vi "Find MBR of Polygon.vi"(0 "Overlay Ref":refnum<k24>, 11 "error in (no error)":errorcluster) -> (3 "Points of Polygon":T1[](array[typedef]) {"Latitude" format="%#_10g"; "Longitude" format="%#_10g"}, 4 "Min Lat":dbl format="%#.6g", 6 "Min Lon":dbl format="%#.6g", 8 "Max Lat":dbl format="%#.6g", 10 "Max Lon":dbl format="%#.6g", 14 "Bearing Between First two Points":dbl, 15 "error out":errorcluster)   [LabVIEW 2014]
uses:
  C:/Robotic Systems/Products/AgFalcon/Software/Ground Station/Data/Mapping DLL/GMap.NET.WindowsForms.dll
  Data/Mapping DLL/GMap.NET.WindowsForms.dll
  Lat Long Conversion/Controls/PointLatLon.ctl
  C:/Robotic Systems/Products/AgFalcon/Software/Ground Station/Data/Mapping DLL/GMap.NET.Core.dll
  Data/Mapping DLL/GMap.NET.Core.dll
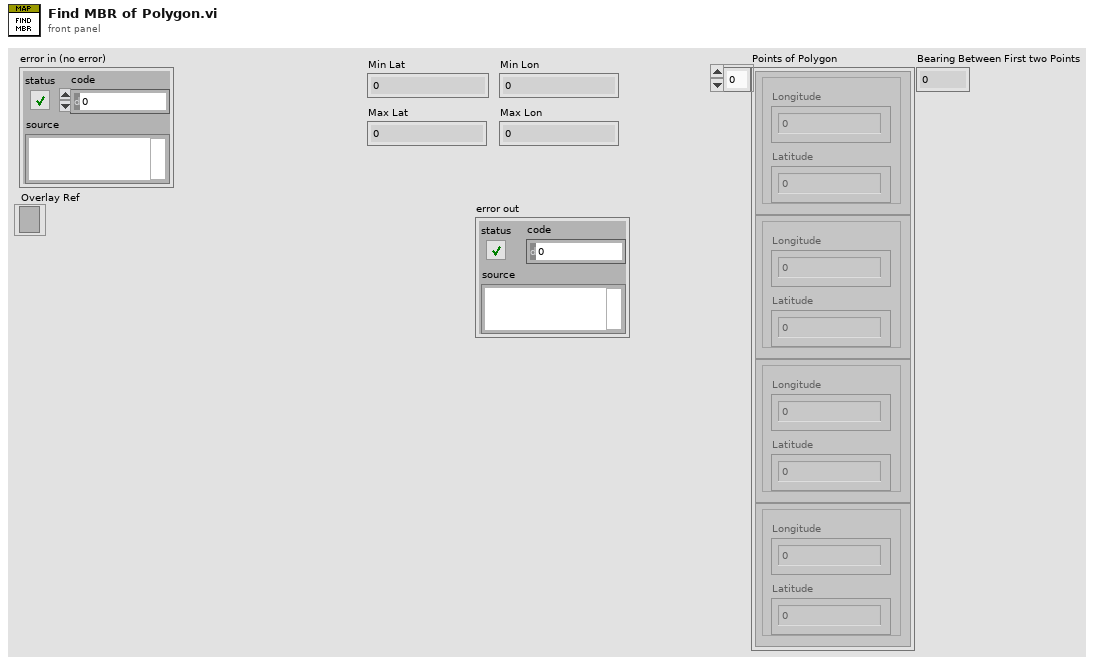
[diagram p1: front panel]
types:
  T1 = typedef "PointLatLon.ctl" = cluster{"Longitude":dbl, "Latitude":dbl}
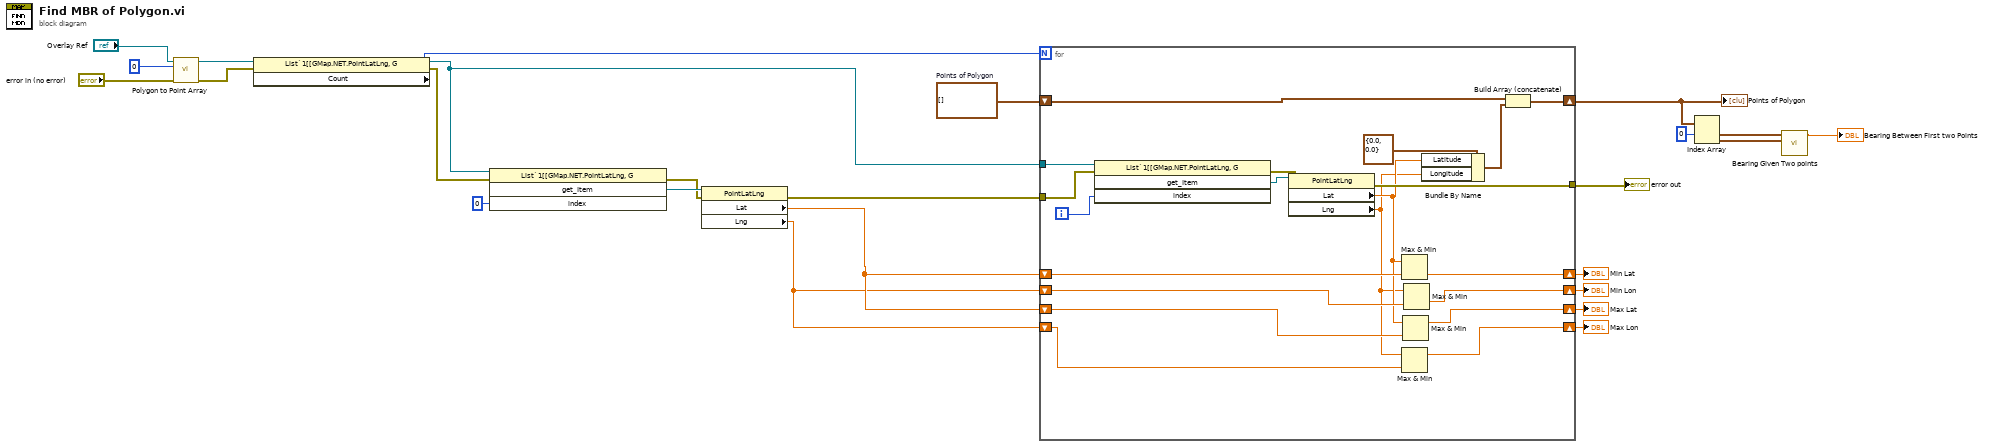
[diagram p0: block diagram]
diagram:
  w6 = T1[] []  # Points of Polygon
  n1 = call "Polygon to Point Array.vi"("error in (no error)"="error in (no error)", "Polygon Index"=0, "Overlay Ref"="Overlay Ref") -> ("error out"=w21:errorcluster, "Points"=w22:refnum<k24>)  [unwired: 7 in]
  n2 = property class="List`1[[GMap.NET.PointLatLng, G"(reference=w22, error in=w21) -> (reference out=w18:refnum<k24>, error out=w19:errorcluster, "Count"=w20:i32)
  n3 = invoke class="List`1[[GMap.NET.PointLatLng, G" method="get_Item"(reference=w18, error in=w19, "index"=0) -> (error out=w15:errorcluster, "get_Item"=w16:refnum<k24>)  [unwired: 1 in, 2 out]
  n4 = property class="PointLatLng"(reference=w16, error in=w15) -> (error out=w12:errorcluster, "Lat"=w14:dbl, "Lng"=w13:dbl)  [unwired: 1 out]
  n5 = for {
    N: w20 -> [_]
    tunnel: w12 -> [w44]
    tunnel: w18 -> [w45]
    shift-right: [w39] -> w11
    shift-left: w14 -> [w40]
    shift-right: [w37] -> w10
    shift-left: w13 -> [w38]
    shift-right: [w34] -> w9
    shift-left: w14 -> [w36]
    shift-right: [w33] -> w8
    shift-left: w13 -> [w35]
    tunnel: [w32] -> w7
    shift-right: [w27] -> w5
    shift-left: w6 -> [w28]
    i -> [w43]
    n6 = invoke class="List`1[[GMap.NET.PointLatLng, G" method="get_Item"(reference=w45, error in=w44, "index"=w43) -> (error out=w41:errorcluster, "get_Item"=w42:refnum<k24>)  [unwired: 1 in, 2 out]
    n7 = property class="PointLatLng"(reference=w42, error in=w41) -> (error out=w32:errorcluster, "Lat"=w30:dbl, "Lng"=w29:dbl)  [unwired: 1 out]
    n8 = Max & Min(x=w30, y=w40) -> (min(x,y)=w39:dbl)  [unwired: 1 out]
    n9 = Max & Min(x=w29, y=w35) -> (max(x,y)=w33:dbl)  [unwired: 1 out]
    n10 = Max & Min(x=w30, y=w36) -> (max(x,y)=w34:dbl)  [unwired: 1 out]
    n11 = Max & Min(x=w29, y=w38) -> (min(x,y)=w37:dbl)  [unwired: 1 out]
    n12 = Bundle By Name(cluster=T1 {"Longitude"=0.0, "Latitude"=0.0} ("Origin Point"), "Latitude"=w30, "Longitude"=w29) -> (w26:T1)
    n13 = Build Array (concatenate)(w28, w26) -> (w27:T1[])
  }
  "Min Lat" <- w11
  "Min Lon" <- w10
  "Max Lat" <- w9
  "Max Lon" <- w8
  "error out" <- w7
  "Points of Polygon" <- w5
  n14 = Index Array(array=w5, index #1=0 ("index")) -> (element #1=w3:T1, element #2=w2:T1)  [unwired: 1 in]
  n15 = call "Bearing Given Two points.vi"("End Point"=w2, "Origin Point"=w3) -> ("Bearing (True North)"=→"Bearing Between First two Points":dbl)  [unwired: 8 in, 1 out]
